vi "Get_Folder_Details.vi"(0 "Path":path, 11 "Error_In":errorcluster) -> (3 "Directory":bool, 4 "Path_Out":path, 6 "Parent_Path":path, 8 "Filename":string, 10 "Size":i64, 15 "Error_Out":errorcluster)   [LabVIEW 2021, in "Custom_Sort_Library.lvlib"]
doc: "This VI get folder details"
uses:
  Custom_Sort_Library.lvlib
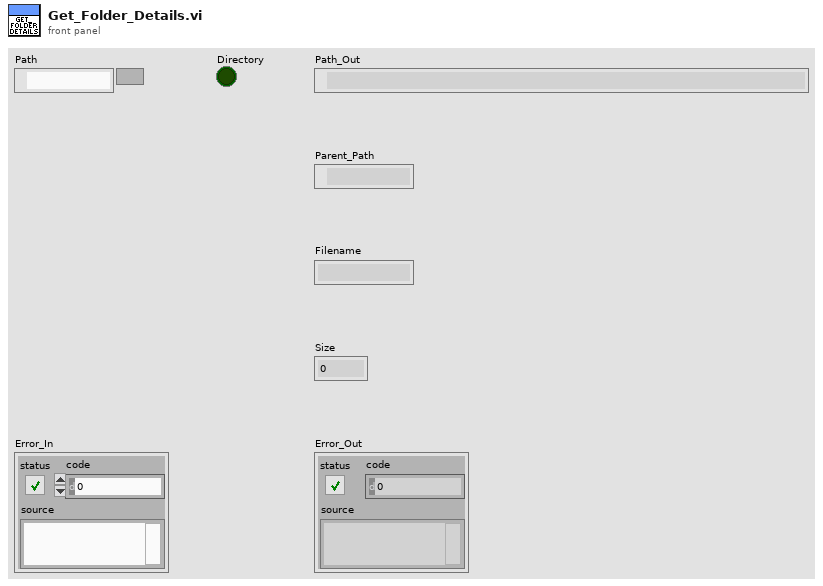
[diagram p1: front panel]
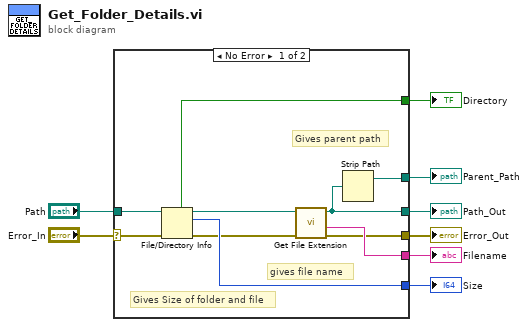
[diagram p0: block diagram]
diagram:
  n1 = case shown="No Error" "Error_In" {
    selector: "Error_In" -> [w16 w20]
    tunnel: "Path" -> [w15 w19]
    tunnel: [w18 _] -> w7
    tunnel: [w17 _] -> w6
    tunnel: [w14 _] -> w4
    tunnel: [w11 w19] -> w3
    tunnel: [w10 w20] -> w2
    tunnel: [w9 _] -> w1
    frame No Error {
      # "Gives parent path"
      # "gives file name"
      # "Gives Size of folder and file"
      n2 = File/Directory Info(path=w15, error in=w16) -> (path out=w12:path, directory=w17:bool, size=w18:i64, error out=w13:errorcluster)  [unwired: 3 out]
      n3 = call <vilib>:"Get File Extension.vi"("error in (no error)"=w13, "file"=w12) -> ("error out"=w10:errorcluster, "filename without extension"=w14:string, "dup file"=w11:path)  [unwired: 5 in, 2 out]
      n4 = Strip Path(path=w11) -> (stripped path=w9:path)  [unwired: 1 out]
    }
    frame Error {
    }
  }
  "Size" <- w7
  "Error_Out" <- w2
  "Path_Out" <- w3
  "Directory" <- w6
  "Filename" <- w4
  "Parent_Path" <- w1
